vi "Set Voltage.vi"(8 "error in":errorcluster, 11 "Acopian in":refnum<class "Acopian.lvclass">) -> (0 "error out":errorcluster, 3 "Acopian out":refnum<class "Acopian.lvclass">)   [LabVIEW 2019, in "Acopian.lvlib" / "Acopian.lvclass"]
uses:
  Library/Acopian.lvclass
  C:/Users/Public/Documents/Development/builds/Instruments/PowerSupply.lvlibp/Library/PowerSupply.lvclass
  Library/Acopian.lvclass/Acopian.ctl
  Accessors/Read Local Resource.vi
  Accessors/Write Local Resource.vi
panel:
  out "read buffer":string
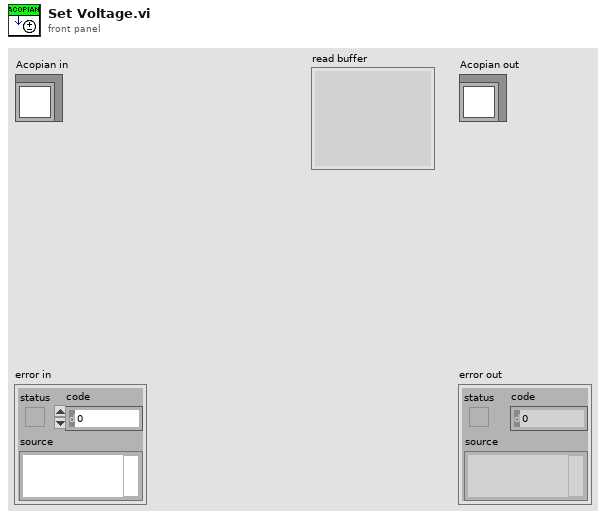
[diagram p1: front panel]
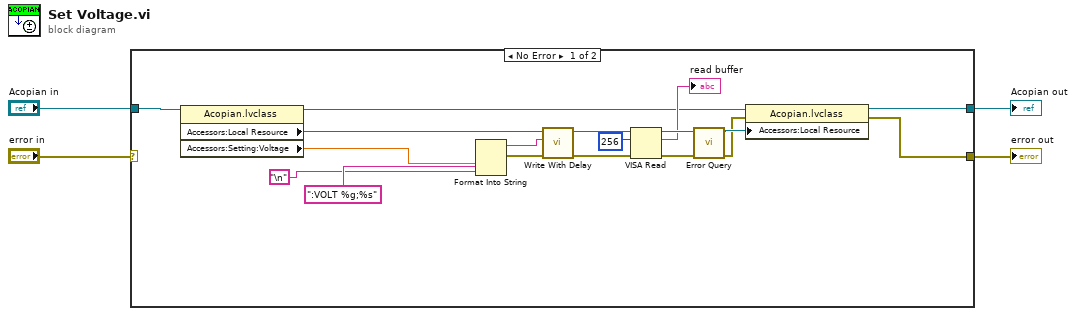
[diagram p0: block diagram]
diagram:
  n1 = case shown="No Error" "error in" {
    selector: "error in" -> [_ w24]
    tunnel: [w17 w24] -> w3
    tunnel: [w21 w23] -> w1
    tunnel: "Acopian in" -> [w22 w23]
    frame No Error {
      n2 = property class="Acopian.lvclass"(reference=w22) -> (reference out=w6:refnum<class "Acopian.lvclass">, "Accessors:Local Resource"=w18:refnum<visa-resource-name>, "Accessors:Setting:Voltage"=w5:dbl)  [unwired: 1 in, 1 out]
      n3 = Format Into String(format string=":VOLT %g;%s" ("Set Voltage"), w5, "\n") -> (resulting string=w16:string, error out=w19:errorcluster)  [unwired: 2 in]
      n4 = call "Write With Delay.vi"("error in"=w19, "write buffer"=w16, "VISA resource name"=w18) -> ("error out"=w12:errorcluster, "VISA resource name out"=w13:refnum<visa-resource-name>)  [unwired: 7 in]
      n5 = VISA Read(VISA resource name=w13, byte count=u32 256, error in (no error)=w12) -> (VISA resource name out=w10:refnum<visa-resource-name>, read buffer=→"read buffer":string, error out=w11:errorcluster)  [unwired: 1 out]
      n6 = call "Error Query.vi"("error in"=w11, "VISA resource in"=w10) -> ("error out"=w8:errorcluster, "VISA resource out"=w9:refnum<visa-resource-name>)  [unwired: 6 in, 2 out]
      n7 = property class="Acopian.lvclass"(reference=w6, error in=w8, "Accessors:Local Resource"=w9) -> (reference out=w21:refnum<class "Acopian.lvclass">, error out=w17:errorcluster)
    }
    frame Error {
    }
  }
  "error out" <- w3
  "Acopian out" <- w1
